vi "reconstruct single image for display.vi"(6 "bidirection?":bool=TRUE, 7 "x fly back pixel":u16, 8 "PXI channel":T1={"Vertical Range (V)"=1.0, "Min Sample Rate"=2208791.906743315, "# of Channels"=1, "Min Record Length"=560, "Number Of Records"=10000, "Trigger Position(%)"=0.0, "act Record Length"=1000, "trigger source"="VAL_EXTERNAL", "PMT2 # of Channels"=1} {"PMT2 # of Channels" min=1 max=8 step=1; "act Record Length" min=0 max=100000 step=1 format="%#.3g"; "Trigger Position(%)" min=0.0 max=100.0 format="%#.3p"; "Number Of Records" min=0 max=1000000 step=1 format="%#.3g"; "Min Record Length" min=0 max=10000 step=1; "# of Channels" min=1 max=8 step=1; "Min Sample Rate" min=0.0 max=100000000.0 format="%#.3p"; "Vertical Range (V)" min=0.0 max=10.0 format="%#.3g"}, 9 "advanced params":T4={"x flyback time(%)"=40.0, "signal offset"=0, "frame time(s)"=0.0, "fetch # per frame"=1, "galvo sampling rate"=0} {"galvo sampling rate" max=100 step=1 format="%#.3g"; "fetch # per frame" max=100 step=1 format="%#.3g"; "frame time(s)" min=0.0 max=10000.0 format="%#.3g"; "signal offset" max=200 format="%#.3g"; "x flyback time(%)" min=0.0 max=200.0 format="%#.3g"}, 10 "basic params":T3={"X pixel #"=200, "X pixel size(um)"=1.0, "Y pixel #"=200, "Y pixel size(um)"=10.0, "line rate(Hz)"=1.0, "stage scan?"=FALSE} {"line rate(Hz)" min=1.0 max=2000.0 format="%#.3g"; "X pixel size(um)" min=0.0 max=10.0 format="%#.3g"; "X pixel #" min=2 max=20480 step=2 format="%#.3g"; "Y pixel size(um)" min=0.0 max=10.0 format="%#.3g"; "Y pixel #" min=2 max=204800 step=2 format="%#.3g"}, 11 "raw data":i16[][](array[numeric])) -> (3 "images":i16[][][](array[numeric]))   [LabVIEW 2015]
uses:
  type def/advanced params.ctl
  type def/basic params.ctl
  type def/PXI control.ctl
  <instrlib>/niScope/Controls/niScope trigger source digital.ctl
panel:
  out "size(s) 6":i32[](array[numeric])
  out "size(s) 4":i32[](array[numeric])
  out "size(s) 5":i32[](array[numeric])
  out "size(s) 3":i32[](array[numeric])
  out "size(s) 2":i32[](array[numeric])
  out "size(s)":i32[](array[numeric])
  in  "index (page)":i32
  out "final image":i16[][](graph)
  out "recombine image":i16[][](graph)
  out "backward direction":i16[][](graph)
  out "forward directon":i16[][](graph)
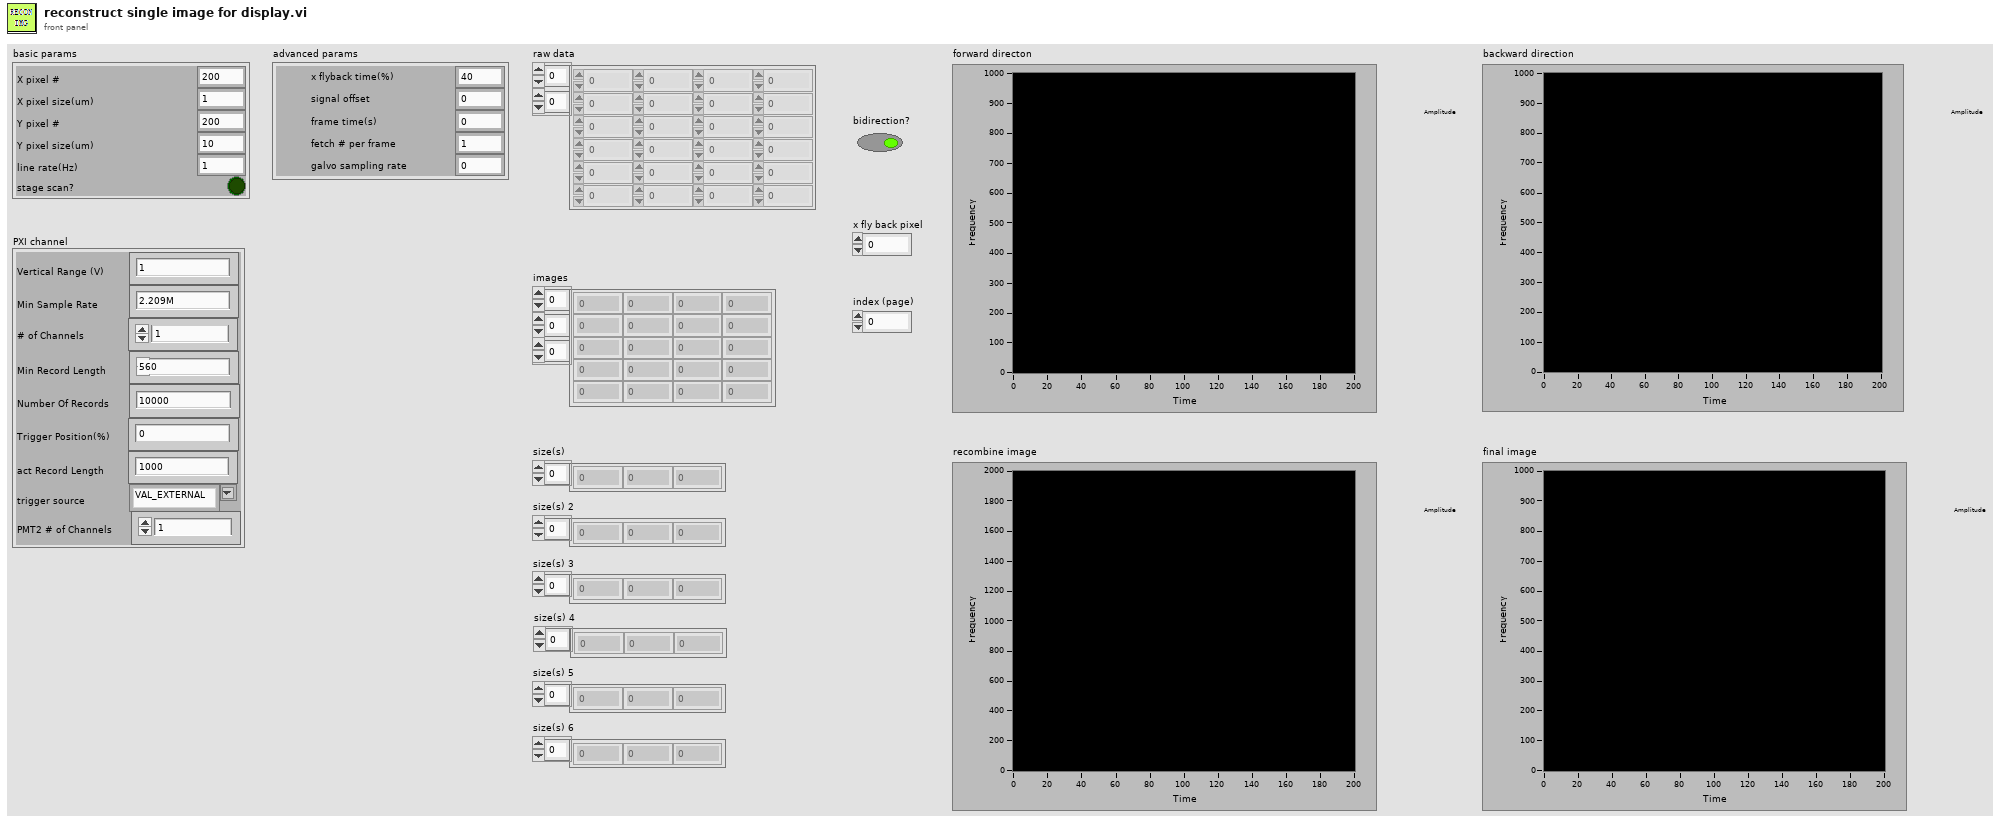
[diagram p1: front panel]
types:
  T1 = typedef "PXI control.ctl" = cluster{"Vertical Range (V)":dbl, "Min Sample Rate":dbl, "# of Channels":u8, "Min Record Length":i32, "Number Of Records":i32, "Trigger Position(%)":dbl, "act Record Length":i32, "trigger source":T2, "PMT2 # of Channels":u8}
  T2 = typedef "niScope trigger source digital.ctl" = string
  T3 = typedef "basic params.ctl" = cluster{"X pixel #":u32, "X pixel size(um)":dbl, "Y pixel #":u32, "Y pixel size(um)":dbl, "line rate(Hz)":dbl, "stage scan?":bool}
  T4 = typedef "advanced params.ctl" = cluster{"x flyback time(%)":dbl, "signal offset":u16, "frame time(s)":dbl, "fetch # per frame":u16, "galvo sampling rate":u32}
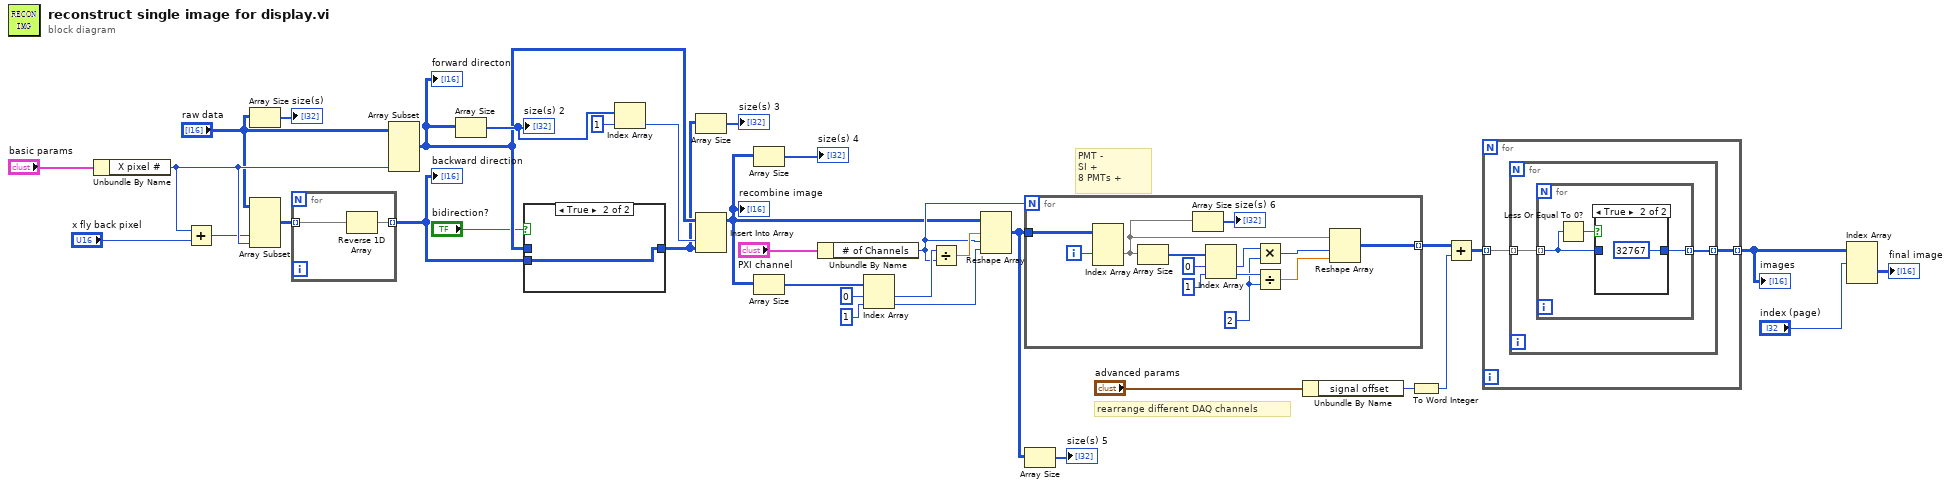
[diagram p0: block diagram]
diagram:
  # "PMT -\nSI +\n8 PMTs +"
  # "rearrange different DAQ channels"
  n1 = Unbundle By Name("basic params") -> ("X pixel #"=w33:u32)
  n2 = Add(x=w33, y="x fly back pixel") -> (x+y=w32:u32)
  n3 = Array Size(array="raw data") -> (size(s)=→"size(s)":i32[])
  n4 = Array Subset(array="raw data", index (col)=w32, length (col)=w33) -> (w31:i16[][])  [unwired: 2 in]
  n5 = for {
    tunnel: w31 -> [w37] mode=indexing
    tunnel: [w36] -> w17 mode=indexing
    n6 = Reverse 1D Array(array=w37) -> (reversed array=w36:i16[])
  }
  "backward direction" <- w17
  n7 = Array Subset(array="raw data", length (col)=w33) -> (w18:i16[][])  [unwired: 3 in]
  "forward directon" <- w18
  n8 = Array Size(array=w18) -> (size(s)=w30:i32[])
  "size(s) 2" <- w30
  n9 = case shown="True" "bidirection?" {
    tunnel: w18 -> [w38 _]
    tunnel: [w38 w39] -> w8
    tunnel: w17 -> [_ w39]
    frame False {
    }
    frame True {
    }
  }
  n10 = Index Array(array=w30, index=1) -> (element=w28:i32)
  n11 = Array Size(array=w8) -> (size(s)=→"size(s) 3":i32[])
  n12 = Insert Into Array(array=w18, index (col)=w28, new element=w8) -> (w1:i16[][])  [unwired: 1 in]
  "recombine image" <- w1
  n13 = Array Size(array=w1) -> (size(s)=→"size(s) 4":i32[])
  n14 = Array Size(array=w1) -> (size(s)=w22:i32[])
  n15 = Unbundle By Name("PXI channel") -> ("# of Channels"=w21:u8)
  n16 = Index Array(array=w22, index #1=0 ("index"), index #2=1 ("index")) -> (element #1=w26:i32, element #2=w23:i32)
  n17 = Divide(x=w26, y=w21) -> (x/y=w27:dbl)
  n18 = Reshape Array(w1, w27, w21, w23) -> (w6:i16[][][])
  n19 = for {
    N: w21 -> [_]
    tunnel: w6 -> [w52]
    tunnel: [w43] -> w3 mode=indexing
    i -> [w42]
    w46 = 2 ("y")
    n20 = Index Array(array=w52, index (dim 1)=w42) -> (element=w40:i16[][])  [unwired: 2 in]
    n21 = Array Size(array=w40) -> (size(s)=w50:i32[])
    n22 = Array Size(array=w40) -> (size(s)=→"size(s) 6":i32[])
    n23 = Index Array(array=w50, index #1=0 ("index (row)"), index #2=1 ("disabled index (col)")) -> (element #1=w45:i32, element #2=w48:i32)
    n24 = Multiply(x=w45, y=w46) -> (x*y=w44:i32)
    n25 = Divide(x=w48, y=w46) -> (x/y=w47:dbl)
    n26 = Reshape Array(w40, w44, w47) -> (w43:i16[][])
  }
  n27 = Array Size(array=w6) -> (size(s)=→"size(s) 5":i32[])
  n28 = Unbundle By Name("advanced params") -> ("signal offset"=w20:u16)
  n29 = To Word Integer(number=w20) -> (16bit integer=w14:i16)
  n30 = Add(x=w3, y=w14) -> (x+y=w11:i16[][][])
  n31 = for {
    tunnel: w11 -> [w54] mode=indexing
    tunnel: [w53] -> w4 mode=indexing
    n32 = for {
      tunnel: w54 -> [w56] mode=indexing
      tunnel: [w55] -> w53 mode=indexing
      n33 = for {
        tunnel: w56 -> [w58] mode=indexing
        tunnel: [w59] -> w55 mode=indexing
        n34 = Less Or Equal To 0?(x=w58) -> (x <= 0?=w57:bool)
        n35 = case shown="True" w57 {
          tunnel: [w60 i16 32767 ("x")] -> w59
          tunnel: w58 -> [w60 _]
          frame False {
          }
          frame True {
          }
        }
      }
    }
  }
  "images" <- w4
  n36 = Index Array(array=w4, index (dim 0)="index (page)") -> (element=→"final image":i16[][])  [unwired: 2 in]
